vi "ListIO.vi"(11 "Project":refnum<vi>) -> (0 "DI/O":string[](array[string]), 1 "AI":string[](array[string]), 2 "AO":string[](array[string]), 3 "DIOPORT":string[](array[string]))   [LabVIEW 2014]
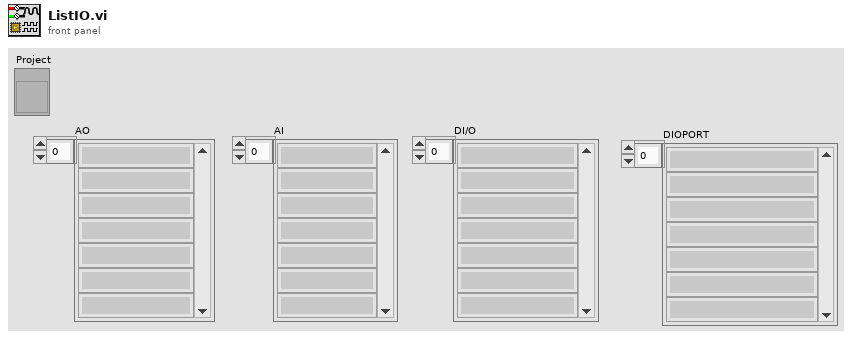
[diagram p1: front panel]
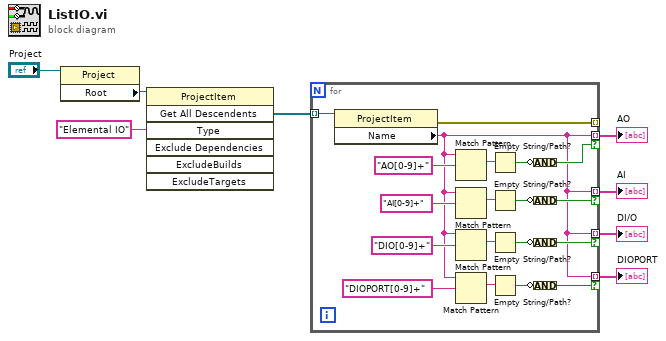
[diagram p0: block diagram]
diagram:
  n1 = property class="Project"(reference="Project") -> ("Root"=w6:refnum<vi>)  [unwired: 1 in, 2 out]
  n2 = invoke class="ProjectItem" method="Get All Descendents"(reference=w6, "Type"="Elemental IO" ("Type String")) -> ("All Descendents"=w7:refnum<vi>[])  [unwired: 5 in, 6 out]
  n3 = for {
    tunnel: w7 -> [w27] mode=indexing
    tunnel: [w10] -> w8 mode=indexing if=w23
    tunnel: [w26] -> _ mode=indexing
    tunnel: [w10] -> w4 mode=indexing if=w15
    tunnel: [w10] -> w3 mode=indexing if=w14
    tunnel: [w10] -> w1 mode=indexing if=w9
    n4 = property class="ProjectItem"(reference=w27) -> (error out=w26:errorcluster, "Name"=w10:string)  [unwired: 1 in, 1 out]
    n5 = Match Pattern(string=w10, regular expression="AO[0-9]+") -> (match substring=w24:string)  [unwired: 1 in, 3 out]
    n6 = Match Pattern(string=w10, regular expression="AI[0-9]+") -> (match substring=w20:string)  [unwired: 1 in, 3 out]
    n7 = Match Pattern(string=w10, regular expression="DIO[0-9]+") -> (match substring=w17:string)  [unwired: 1 in, 3 out]
    n8 = Match Pattern(string=w10, regular expression="DIOPORT[0-9]+") -> (match substring=w12:string)  [unwired: 1 in, 3 out]
    n9 = Empty String/Path?(string/path=w24) -> (empty?=w22:bool)
    n10 = Empty String/Path?(string/path=w20) -> (empty?=w21:bool)
    n11 = Empty String/Path?(string/path=w17) -> (empty?=w16:bool)
    n12 = Empty String/Path?(string/path=w12) -> (empty?=w13:bool)
    n13 = Compound Arithmetic op=AND(invert w22) -> (w23:bool)
    n14 = Compound Arithmetic op=AND(invert w21) -> (w15:bool)
    n15 = Compound Arithmetic op=AND(invert w16) -> (w14:bool)
    n16 = Compound Arithmetic op=AND(invert w13) -> (w9:bool)
  }
  "AO" <- w8
  "AI" <- w4
  "DI/O" <- w3
  "DIOPORT" <- w1
